vi "ni5660 Sub Get Multi-Span Settings.vi"(0 "receiver info in":T2, 11 "error in (no error)":errorcluster) -> (4 "receiver info out":T2, 6 "multispan settings":T1 {"df" format="%.2f"; "fc adjustment" format="%.2f"; "segment size" format="%.2f"; "frequency shifts" format="%.2f"}, 10 "found":bool, 15 "error out":errorcluster)   [LabVIEW 2011]
uses:
  <vilib>/addons/Modulation/niScope/controls/mod_Modulation Settings.ctl
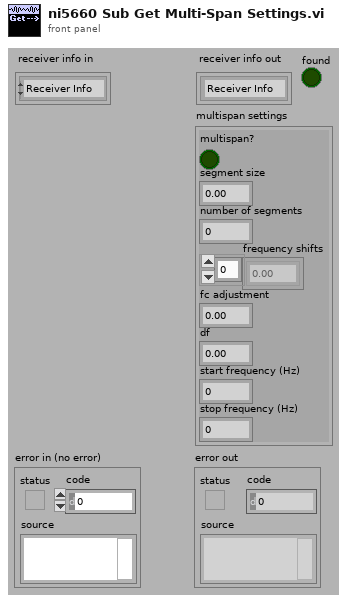
[diagram p1: front panel]
types:
  T1 = cluster{"multispan?":bool, "segment size":dbl, "number of segments":i32, "frequency shifts":dbl[], "fc adjustment":dbl, "df":dbl, "start frequency (Hz)":dbl, "stop frequency (Hz)":dbl}
  T2 = typedef "mod_Modulation Settings.ctl" = cluster{enum16{"Receiver Info"}, variant}
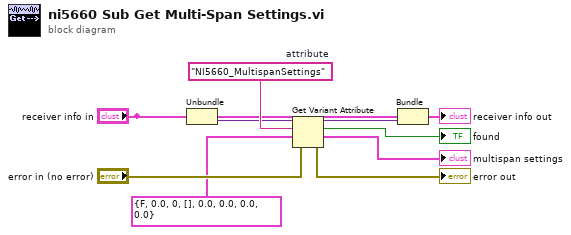
[diagram p0: block diagram]
diagram:
  w10 = "NI5660_MultispanSettings"  # attribute
  n1 = Unbundle("receiver info in") -> (w6:variant)  [unwired: 1 out]
  n2 = Get Variant Attribute(Variant=w6, name=w10, default value (empty Variant)=T1 {"multispan?"=FALSE, "segment size"=0.0, "number of segments"=0, "frequency shifts"=[], "fc adjustment"=0.0, "df"=0.0, "start frequency (Hz)"=0.0, "stop frequency (Hz)"=0.0} ("multispan settings"), error in="error in (no error)") -> (duplicate Variant=w5:variant, found=→"found":bool, value=→"multispan settings":T1, error out=→"error out":errorcluster)
  n3 = Bundle(cluster="receiver info in", w5) -> (→"receiver info out":T2)  [unwired: 1 in]
